vi "Car_ClassCast.vi"(11 "Car:Car in":refnum<class>) -> (3 "Car:Car out":refnum<class "Car.lvclass">)   [LabVIEW 2021, in "Car.lvlib" / "Car.lvclass"]
uses:
  Car.lvclass
  Car.lvclass/Car.ctl
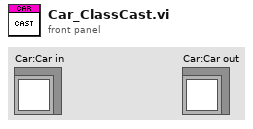
[diagram p1: front panel]
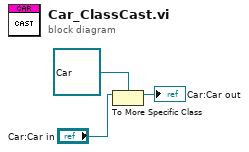
[diagram p0: block diagram]
diagram:
  n1 = To More Specific Class(target class=refnum<class "Car.lvclass"> refnum ("reference in"), reference="Car:Car in") -> (specific class reference=→"Car:Car out":refnum<class "Car.lvclass">)  [unwired: 1 in, 1 out]
